vi "XML - Evaluate Tx Imported Channels.vi"(8 "error in (no error)":errorcluster, 10 "Channel Info Array":T1[](array[typedef]) {"Data Type" items=["U8", "U16", "U32", "U64", "I8", "I16", "I32", "I64", "SGL", "DBL", "EXT"]}, 11 "Node Ptr in":u64 format="%.0x") -> (0 "error out":errorcluster, 2 "Invalid Channels":string[](array[string]), 3 "Node Ptr out":u64 format="%.0x")   [LabVIEW 2019]
uses:
  Types/XML/XML - Channel.ctl
  <vilib>/NI VeriStand/Custom Device API/Custom Device Item Ref.ctl
  Shared/Constants.vi
  <vilib>/NI VeriStand/Custom Device Tools/Custom Device Utility Library/NI VeriStand - Search for Item by GUID.vi
  <vilib>/NI VeriStand/Custom Device Tools/Custom Device Utility Library/Custom Device Utility Library.lvlib
  <vilib>/NI VeriStand/Custom Device API/Custom Device API.lvlib
  Property Accessors/Shared Packet Accessors.lvlib
  Shared/UDP-Custom-Device Shared.lvlib
  UDP-Custom-Device System Explorer.lvlib
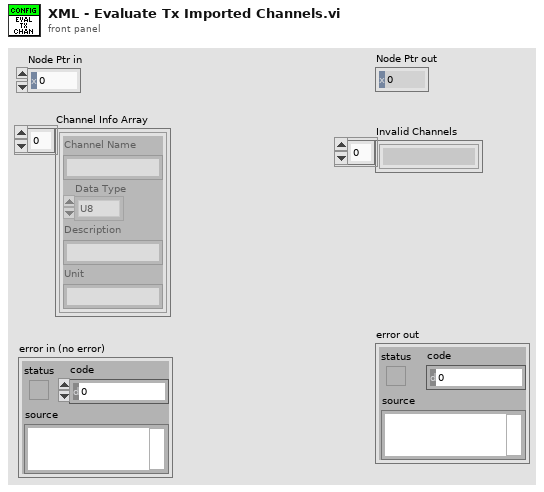
[diagram p1: front panel]
types:
  T1 = typedef "UDP-Custom-Device System Explorer.lvlib/XML - Channel.ctl" = cluster{"Channel Name":string, "Data Type":u16, "Description":string, "Unit":string}
  T2 = typedef "Custom Device API.lvlib/Custom Device Item Ref.ctl" = u64
  T3 = typedef "Custom Device API.lvlib/Custom Device Item Info.ctl" = cluster{"Name":string, "Is Channel":bool, "GUID":string, "Is Waveform":bool}
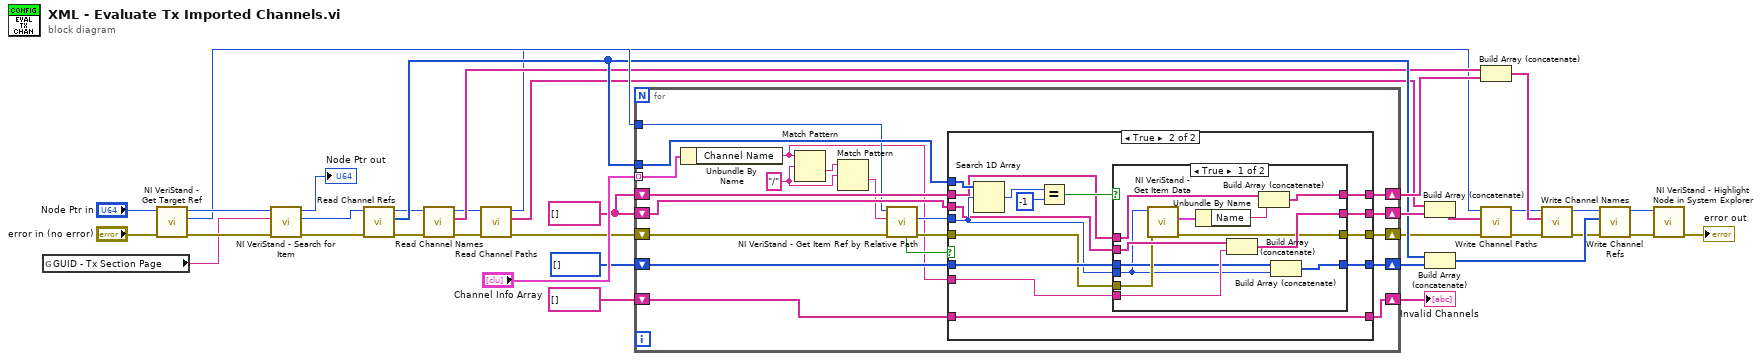
[diagram p0: block diagram]
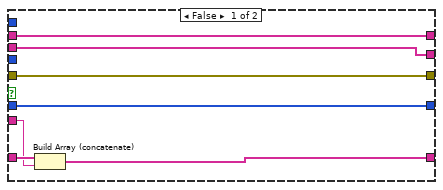
[diagram p2: hidden frame]
diagram:
  w32 = string[] []
  n1 = global read "Constants.vi" "GUID - Tx Section Page"() -> (w1:string)
  n2 = call <vilib>:"NI VeriStand - Get Target Ref.vi"("error in"="error in (no error)", "Item Ref in"="Node Ptr in") -> ("error out"=w26:errorcluster, "Target Ref"=w23:T2, "Item Ref out"=w24:T2)  [unwired: 6 in, 1 out]
  n3 = call-poly <vilib>:"NI VeriStand - Search for Item.vi"("error in"=w26, "Item GUID"=w1, "Section Ref in"=w24) -> ("error out"=w20:errorcluster, "Item Ref"=w22:T2, "Section Ref out"=→"Node Ptr out":T2)  [unwired: 5 in, 1 out]
  n4 = call "Read Channel Refs.vi"("error in (no error)"=w20, "Node Ptr"=w22) -> ("error out"=w18:errorcluster, "Dependent Node Refs"=w21:T2[], "Node Ptr out"=w19:T2)  [unwired: 7 in]
  n5 = call "Read Channel Names.vi"("error in (no error)"=w18, "Node Ptr"=w19) -> ("error out"=w15:errorcluster, "Channel Names"=w17:string[], "Node Ptr out"=w16:T2)  [unwired: 7 in]
  n6 = call "Read Channel Paths.vi"("error in (no error)"=w15, "Node Ptr"=w16) -> ("error out"=w14:errorcluster, "Channel Paths"=w13:string[], "Node Ptr out"=w9:T2)  [unwired: 7 in]
  n7 = for {
    tunnel: "Channel Info Array" -> [w57] mode=indexing
    shift-right: [w56] -> w8
    shift-left: w14 -> [w46]
    shift-right: [w54] -> w35
    shift-left: string[] [] -> [w55]
    tunnel: w21 -> [w53]
    shift-right: [w51] -> w31
    shift-left: T2[] [] -> [w52]
    shift-right: [w49] -> w30
    shift-left: w32 -> [w50]
    shift-right: [w47] -> w29
    shift-left: w32 -> [w48]
    tunnel: w23 -> [w44]
    w39 = "/" ("regular expression")
    n8 = Unbundle By Name(w57) -> ("Channel Name"=w41:string)
    n9 = Match Pattern(string=w41, regular expression=w39) -> (after substring=w40:string)  [unwired: 1 in, 3 out]
    n10 = Match Pattern(string=w40, regular expression=w39) -> (after substring=w38:string)  [unwired: 1 in, 3 out]
    n11 = call <vilib>:"NI VeriStand - Get Item Ref by Relative Path.vi"("error in"=w46, "Relative Item Path"=w38, "Section Ref in"=w44) -> ("error out"=w45:errorcluster, "Item Ref"=w43:T2, "Found"=w42:bool)  [unwired: 5 in, 1 out]
    n12 = case shown="True" w42 {
      tunnel: w45 -> [w61 w71]
      tunnel: [w61 w66] -> w56
      tunnel: w55 -> [w64 w79]
      tunnel: w41 -> [w63 w65]
      tunnel: [w62 w79] -> w54
      tunnel: w53 -> [_ w78]
      tunnel: w43 -> [_ w73]
      tunnel: w52 -> [w60 w74]
      tunnel: [w60 w72] -> w51
      tunnel: w50 -> [w59 w70]
      tunnel: [w59 w69] -> w49
      tunnel: w48 -> [w58 w68]
      tunnel: [w58 w67] -> w47
      frame False {
        n13 = Build Array (concatenate)(w64, w63) -> (w62:string[])
      }
      frame True {
        n14 = Search 1D Array(1D array=w78, element=w73) -> (index of element=w77:i32)  [unwired: 1 in]
        n15 = Equal?(x=w77, y=-1) -> (x = y?=w75:bool)
        n16 = case shown="True" w75 {
          tunnel: w74 -> [w82 w94]
          tunnel: w73 -> [w81 _]
          tunnel: [w80 w94] -> w72
          tunnel: w71 -> [w88 w95]
          tunnel: w70 -> [w84 w93]
          tunnel: [w83 w93] -> w69
          tunnel: w68 -> [w89 w92]
          tunnel: [w90 w92] -> w67
          tunnel: [w87 w95] -> w66
          tunnel: w65 -> [w91 _]
          frame True {
            n17 = call <vilib>:"NI VeriStand - Get Item Data.vi"("error in (no error)"=w88, "Item Ref in"=w81) -> ("error out"=w87:errorcluster, "Item Info"=w86:T3)  [unwired: 6 in, 2 out]
            n18 = Unbundle By Name(w86) -> ("Name"=w85:string)
            n19 = Build Array (concatenate)(w89, w91) -> (w90:string[])
            n20 = Build Array (concatenate)(w84, w85) -> (w83:string[])
            n21 = Build Array (concatenate)(w82, w81) -> (w80:T2[])
          }
          frame False {
          }
        }
      }
    }
  }
  "Invalid Channels" <- w35
  n22 = Build Array (concatenate)(w13, w29) -> (w2:string[])
  n23 = Build Array (concatenate)(w21, w31) -> (w12:T2[])
  n24 = Build Array (concatenate)(w17, w30) -> (w7:string[])
  n25 = call "Write Channel Paths.vi"("error in (no error)"=w8, "Channel Paths"=w2, "Node Ptr"=w9) -> ("error out"=w4:errorcluster, "Node Ptr out"=w6:T2)  [unwired: 7 in]
  n26 = call "Write Channel Names.vi"("error in (no error)"=w4, "Channel Names"=w7, "Node Ptr"=w6) -> ("error out"=w3:errorcluster, "Node Ptr out"=w5:T2)  [unwired: 7 in]
  n27 = call "Write Channel Refs.vi"("error in (no error)"=w3, "Dependent Node Refs"=w12, "Node Ptr"=w5) -> ("error out"=w11:errorcluster, "Node Ptr out"=w10:T2)  [unwired: 7 in]
  n28 = call <vilib>:"NI VeriStand - Highlight Node in System Explorer.vi"("error in (no error)"=w11, "Item Ref in"=w10) -> ("error out"=→"error out":errorcluster)  [unwired: 8 in, 1 out]
